vi "总磷氨氮测量流程.vi"(10 "量程模式":T1, 11 "参数":T2={"站号"=1, "量程切换"=enum."AUTO", "控制命令"=enum."启动测量", "模式设置"=enum."待机", "测量间隔"=0} {"站号" items=["总磷"=1, "总氮"=2]}) -> ()   [LabVIEW 2016, in "斯坦道仪器.lvlib"]
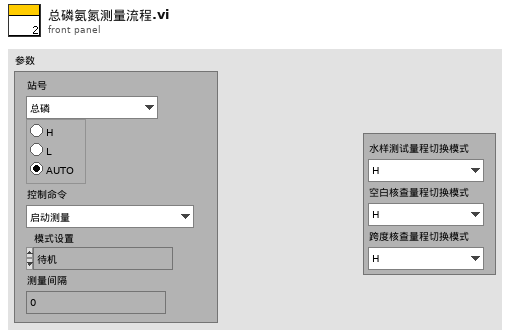
[diagram p1: front panel]
types:
  T1 = cluster{"水样测试量程切换模式":enum16{"H", "L", "AUTO"}, "空白核查量程切换模式":enum16{"H", "L", "AUTO"}, "跨度核查量程切换模式":enum16{"H", "L", "AUTO"}}
  T2 = cluster{"站号":u16, "量程切换":enum32{"H", "L", "AUTO"}, "控制命令":enum16{"启动测量", "标样核查", "零点核查", "跨度核查", "空白测试", "平行样测试", "加标回收", "空白校准", "标样校准", "初始化（清洗）", "停止测试", "仪器重启", "校时", "模式设置", "测量间隔设置"}, "模式设置":enum16{"待机", "连续模式", "周期模式", "定点模式", "受控模式", "手动模式"}, "测量间隔":u16}
  T3 = enum16{"初始化", "通电", "参数1启动", "等待参数1测试完成", "参数1测试完成", "参数1存储数据", "参数2启动", "等待参数2测试完成", "参数2测试完成", "参数2存储数据", "断电", "结束"}
  T4 = cluster{"时间标识":timestamp, "设备":string, "日志信息":string, "流程参数":string}
  T5 = cluster{"时间标识":timestamp, "监测值":sgl, "单位":u16, "数据标识":string, "因子编码":u32, "标样参考值":sgl, "F0":sgl, "F1":sgl, "F2":sgl, "F3":sgl, "F4":sgl, "F5":sgl, "F6":sgl, "F7":sgl, "X":sgl, "温度":sgl, "湿度":sgl, "量程标识":string}
  T6 = enum16{"维护数据", "水样测试", "标样核查", "零点核查", "跨度核查", "空白测试", "平行样测试", "加标回收", "空白校准", "标样校准", "初始化（清洗）"}
  T7 = cluster{"系统时间":timestamp, "工作状态":enum16{"空闲", "水样测试", "标样核查", "零点核查", "跨度核查", "空白测试", "平行样测试", "加标回收", "空白校准", "标样校准", "初始化（清洗）"}, "测量模式":enum16{"待机", "连续模式", "周期模式", "定点模式", "受控模式", "手动模式"}, "告警代码":enum16{"无告警", "缺试剂告警", "缺水样告警", "缺蒸馏水告警", "缺标液告警", "仪表漏液告警", "标定异常告警", "超量程告警", "加热异常", "低试剂预警", "超上限告警", "超下限告警", "仪表内部其他异常", "滴定异常告警", "电极异常告警", "量程切换告警", "参数设置告警", "PH电极电位异常", "电导率电极异常", "浊度光度异常", "溶解氧电极异常", "溶解氧光强异常", "温度异常告警", "PH异常告警", "溶解氧异常告警", "电导率异常告警", "浊度异常告警", "叶绿素异常告警", "藻密度异常告警", "蓝绿藻异常告警", "ORP异常告警", "氨氮异常告警", "清洁刷异常告警", "SD卡异常告警", "蓝牙异常告警", "Wifi异常告警", "流程异常告警"}, "故障代码":enum16{"无故障", "电机故障", "温度故障", "通讯故障", "滴定故障"}, "日志代码":u16, "软件版本":u16, "F0":sgl, "F1":sgl, "F2":sgl, "F3":sgl, "T":sgl, "H":sgl, "id":u16, "flowid":u16, "量程":u16}
  T8 = enum16{"启动测量", "标样核查", "零点核查", "跨度核查", "空白测试", "平行样测试", "加标回收", "空白校准", "标样校准", "初始化（清洗）", "停止测试", "仪器重启", "校时", "模式设置", "测量间隔设置"}
  T9 = enum16{"空闲", "水样测试", "标样核查", "零点核查", "跨度核查", "空白测试", "平行样测试", "加标回收", "空白校准", "标样校准", "初始化（清洗）"}
  T10 = cluster{"时间标识":timestamp, "监测值":sgl, "单位":u16, "数据标识":string, "因子编码":u32, "标样参考值":sgl, "F0":sgl, "F1":sgl, "F2":sgl, "F3":sgl, "温度":sgl, "湿度":sgl, "量程标识":string}
  T11 = cluster{"因子编码":u32, "单位":u16, "标样参考值":sgl, "水样数据时间":timestamp, "水样实测值":sgl, "水样数据标识":string, "标样数据时间":timestamp, "标样实测值":sgl, "标样数据标识":string, "空白数据时间":timestamp, "空白实测值":sgl, "空白数据标识":string, "零点核查数据时间":timestamp, "零点核查实测值":sgl, "零点核查数据标识":string, "跨度核查数据时间":timestamp, "跨度核查实测值":sgl, "跨度核查数据标识":string, "加标回收数据时间":timestamp, "加标回收实测值":sgl, "加标回收数据标识":string, "平行样数据时间":timestamp, "平行样实测值":sgl, "平行样数据标识":string, "F0":sgl, "F1":sgl, "F2":sgl, "F3":sgl, "F4":sgl, "F5":sgl, "F6":sgl, "F7":sgl, "温度":sgl, "湿度":sgl, "X值":sgl}
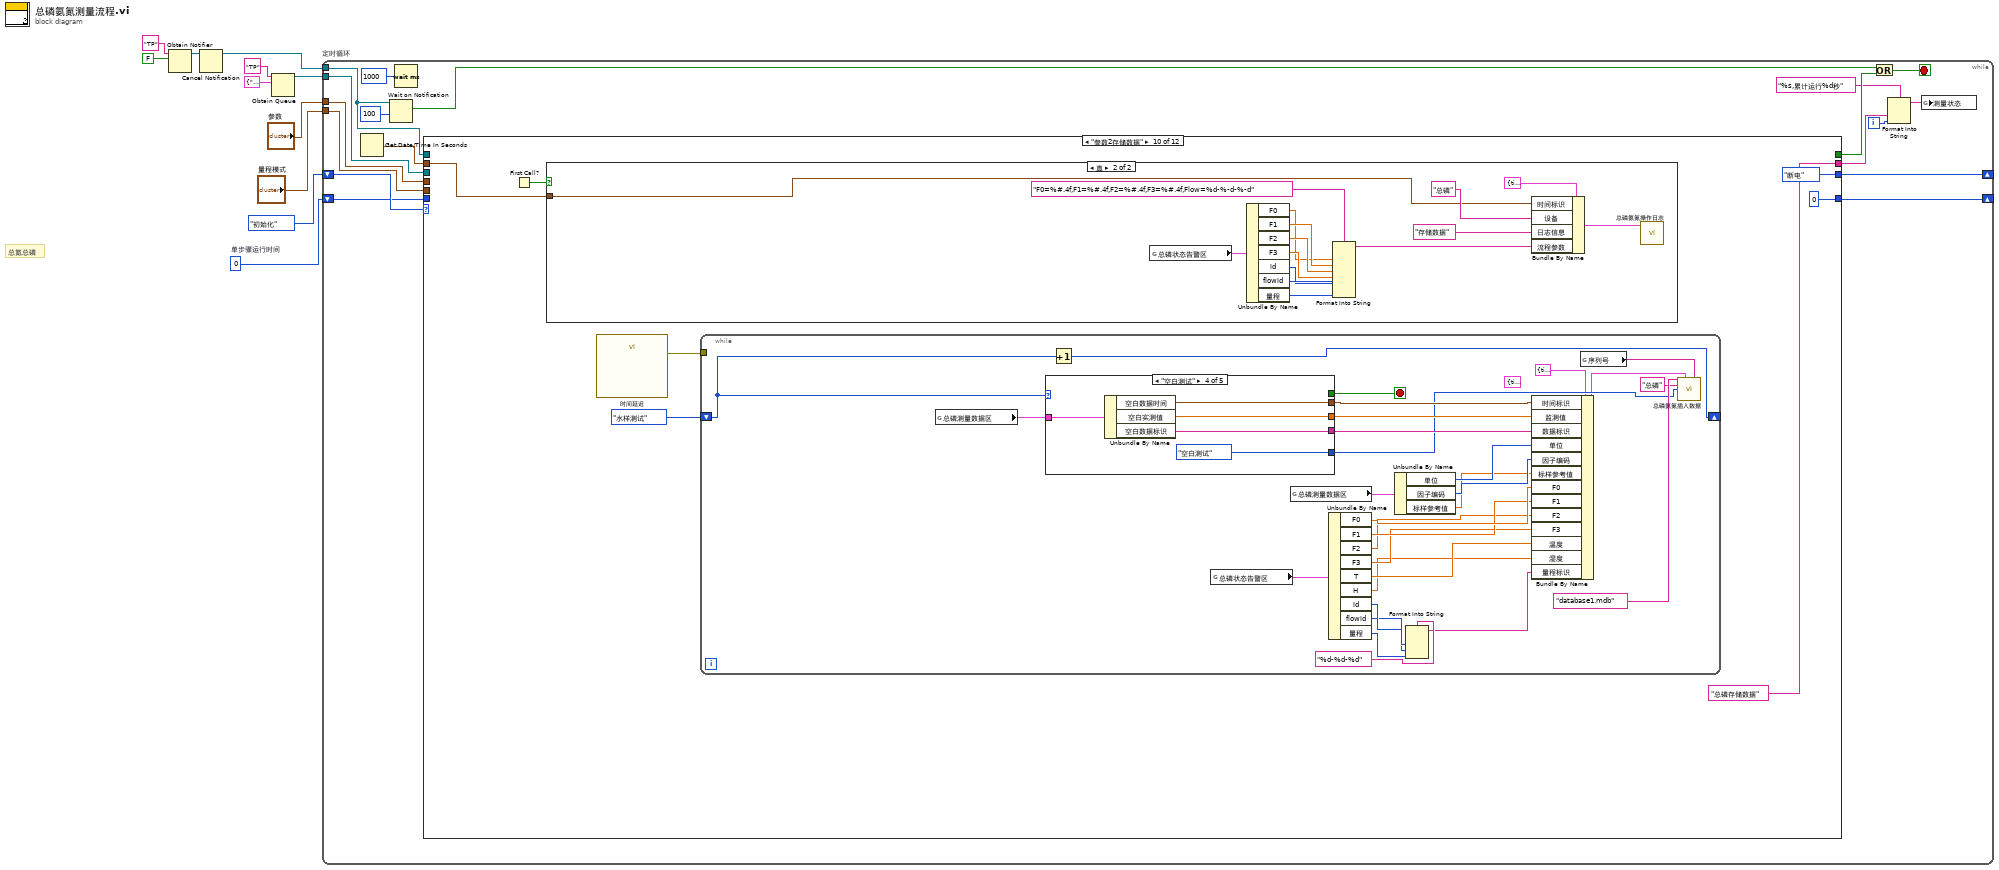
[diagram p0: block diagram]
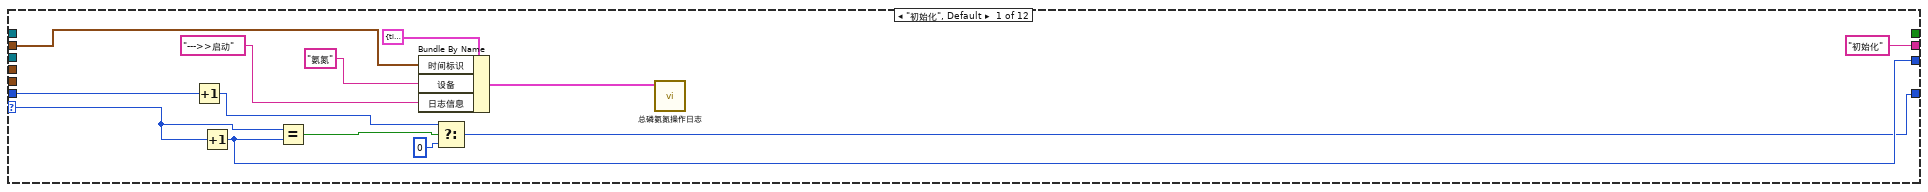
[diagram p2: hidden frame]
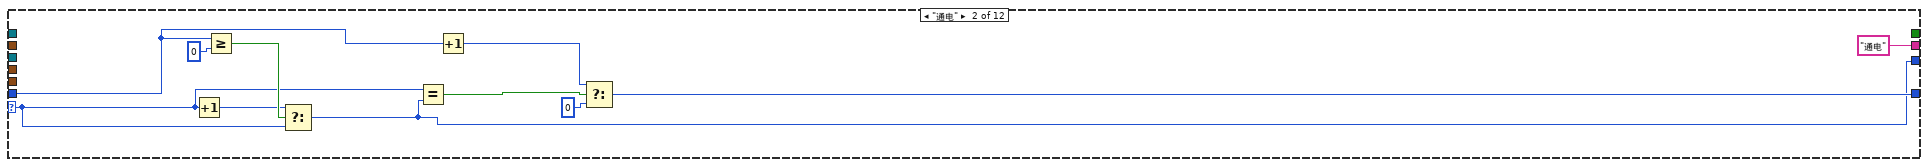
[diagram p3: hidden frame]
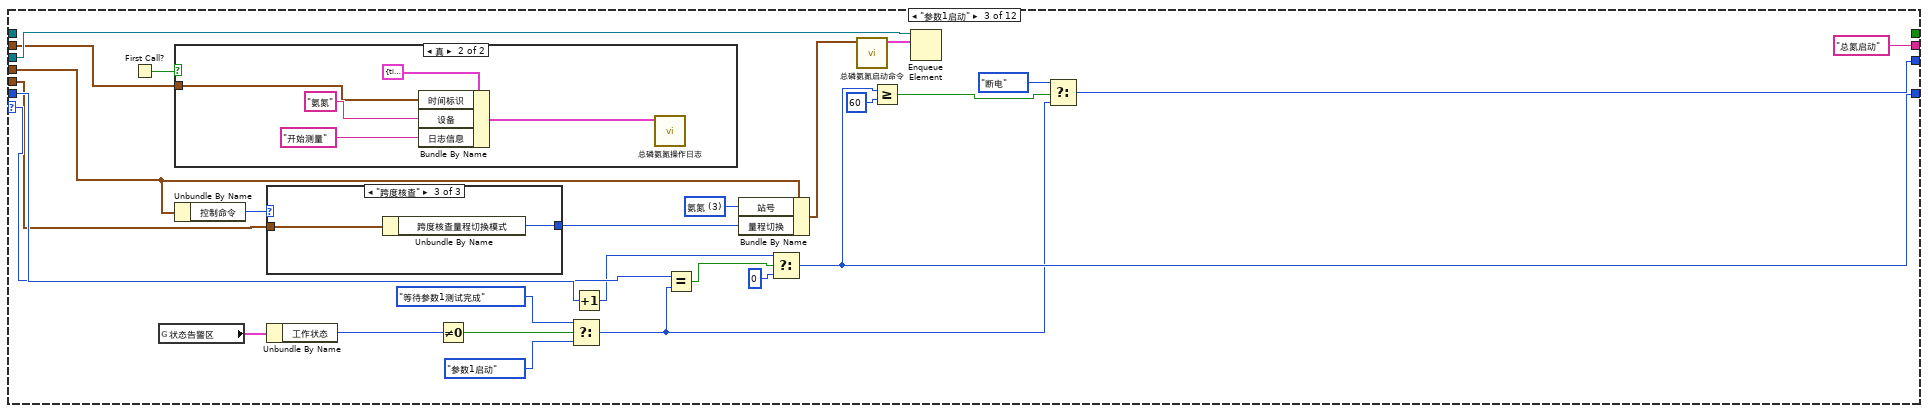
[diagram p4: hidden frame]
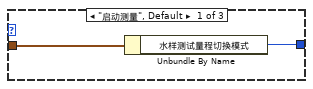
[diagram p5: hidden frame]
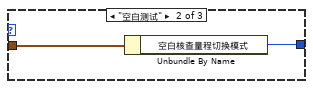
[diagram p6: hidden frame]
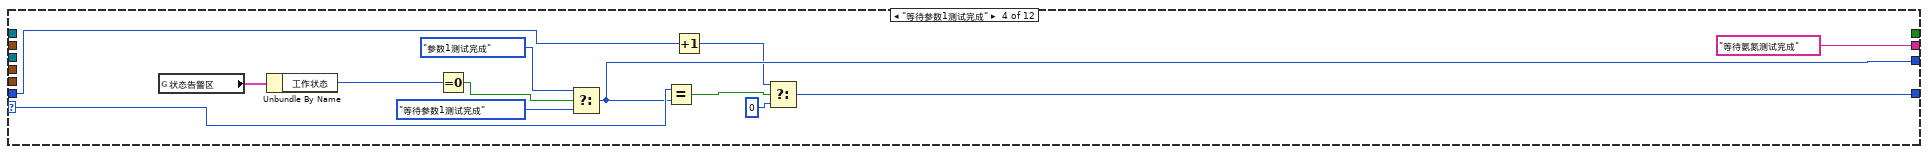
[diagram p8: hidden frame]
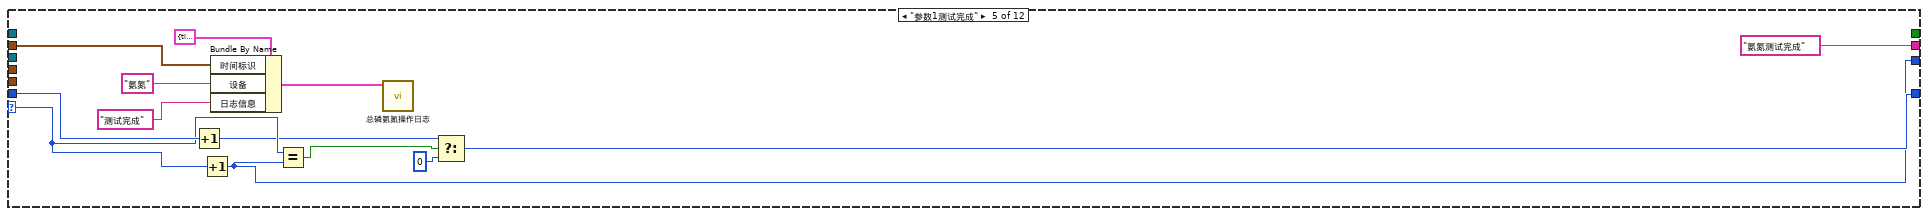
[diagram p9: hidden frame]
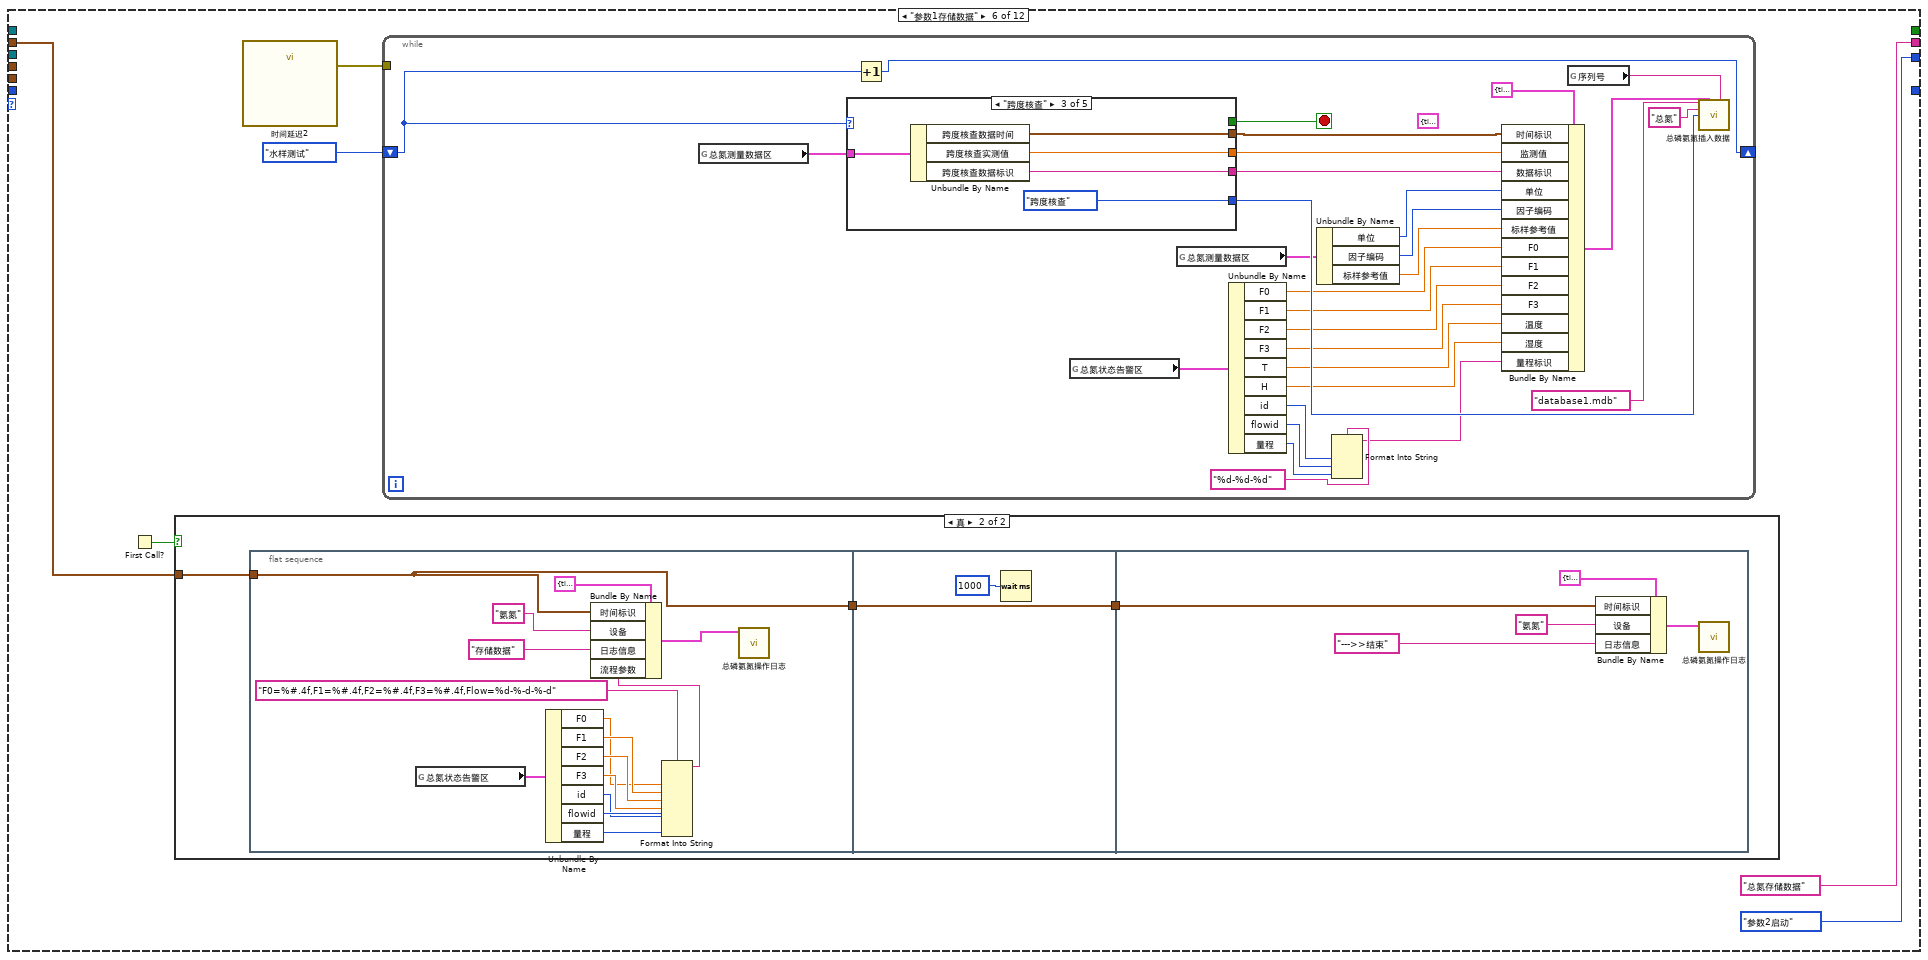
[diagram p10: hidden frame]
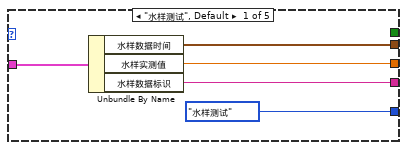
[diagram p11: hidden frame]
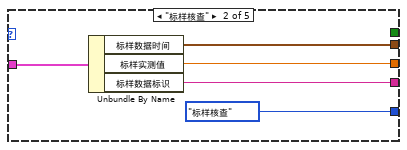
[diagram p12: hidden frame]
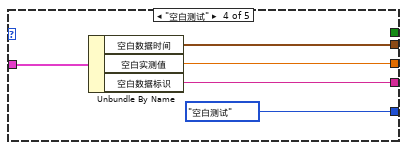
[diagram p13: hidden frame]
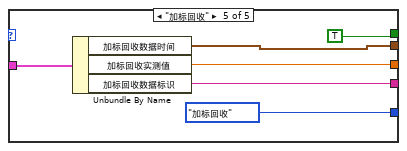
[diagram p14: hidden frame]
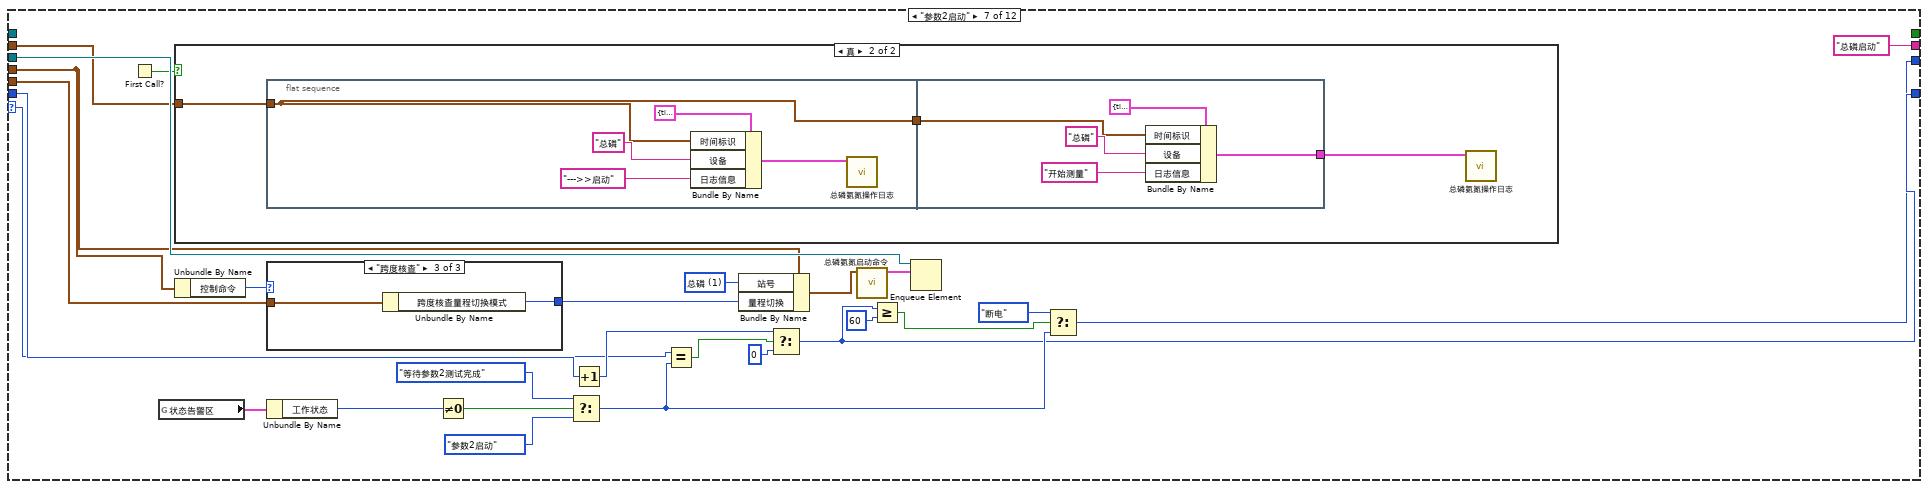
[diagram p16: hidden frame]
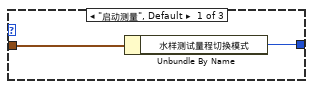
[diagram p17: hidden frame]
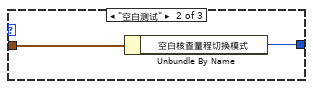
[diagram p18: hidden frame]
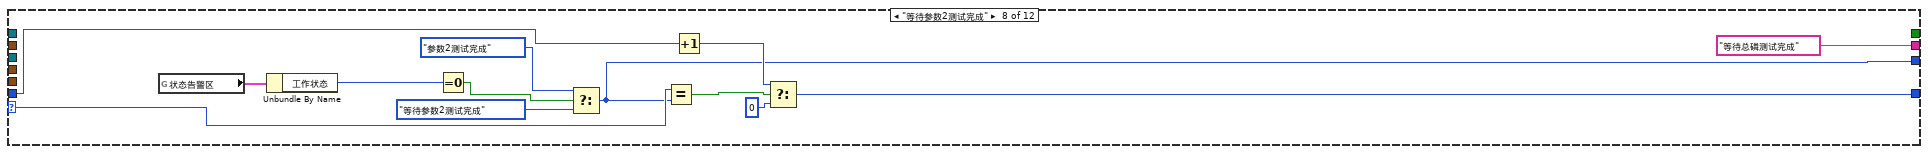
[diagram p20: hidden frame]
diagram:
  w7 = 0  # 单步骤运行时间
  # "总氮总磷"
  n1 = Obtain Notifier(name (unnamed)="TP" ("名称（未命名）"), notification data type=FALSE) -> (notifier out=w4:refnum<notifier>)  [unwired: 2 in, 2 out]
  n2 = Cancel Notification(0:w4) -> (8:w3:refnum<notifier>)  [unwired: 1 in, 2 out]
  n3 = Obtain Queue(name (unnamed)="TP" ("名称（未命名）"), element data type=cluster{"命令":string, "data":variant} {"命令"="", "data"=variant}) -> (queue out=w8:refnum<queue>)  [unwired: 3 in, 2 out]
  n4 = while "定时循环" {
    shift-right: [w28] -> _
    shift-left: T3."初始化" ("枚举") -> [w29]
    tunnel: w8 -> [w27]
    shift-right: [w25] -> _
    shift-left: w7 -> [w26]
    tunnel: w3 -> [w24]
    tunnel: "参数" -> [w19]
    tunnel: "量程模式" -> [w13]
    i -> [w15]
    stop <- w20 stop-if-true
    n5 = Get Date/Time In Seconds() -> (seconds since 1Jan1904=w17:timestamp)
    n6 = Wait on Notification(notifier=w24, timeout in ms (-1)=100 ("超时毫秒(-1)")) -> (notification=w21:bool)  [unwired: 2 in, 3 out]
    n7 = Wait (ms)(milliseconds to wait=u32 1000 ("等待时间（毫秒）")) -> ()  [unwired: 1 out]
    n8 = case shown="\"参数2存储数据\"" w29 {
      selector: w29 -> [w40 w47 w75 w99 w114 _ w219 w255 w271 _ w358 _]
      tunnel: [_ _ _ _ _ _ _ _ _ _ _ TRUE] -> w22
      tunnel: [w41 w46 w54 w98 w113 T3."参数2启动" ("枚举") w204 w253 w269 T3."断电" ("枚举") w357 T3."结束" ("枚举")] -> w28
      tunnel: w27 -> [_ _ w80 _ _ _ w227 _ _ _ _ w370]
      tunnel: w26 -> [w42 w48 w76 w101 w115 _ w220 w256 w272 _ w360 _]
      tunnel: [w38 w49 w59 w100 w116 _ w205 w254 w270 0 ("t") w359 0 ("t")] -> w25
      tunnel: w24 -> [_ _ _ _ _ _ _ _ _ _ _ w369]
      tunnel: w19 -> [_ _ w63 _ _ _ w213 _ _ _ _ _]
      tunnel: w17 -> [w31 _ w68 _ w106 w123 w218 _ w264 w281 _ w363]
      tunnel: ["初始化" ("输入 1") "通电" ("输入 1") "总氮启动" ("输入 1") "等待氨氮测试完成" ("输入 1") "氨氮测试完成" ("输入 1") "总氮存储数据" ("输入 1") "总磷启动" ("输入 1") "等待总磷测试完成" ("输入 1") "总磷测试完成" ("输入 1") "总磷存储数据" ("输入 1") "断电" ("输入 1") "结束" ("输入 1")] -> w14
      tunnel: w13 -> [_ _ w61 _ _ _ w211 _ _ _ _ _]
      frame "初始化", Default {
        n9 = Increment(x=w42) -> (x+1=w36:i32)
        n10 = Increment(x=w40) -> (x+1=w41:T3)
        n11 = Equal?(x=w40, y=w41) -> (x = y?=w39:bool)
        n12 = Bundle By Name(cluster=T4 {"时间标识"=timestamp(0 s since 1904-01-01), "设备"="", "日志信息"="", "流程参数"=""} ("data in"), "时间标识"=w31, "设备"="氨氮", "日志信息"="--->>启动") -> (w35:T4)
        n13 = Select(t=w36, s=w39, f=0 ("t")) -> (s? t:f=w38:i32)
        n14 = call "总磷氨氮操作日志.vi"("data in"=w35) -> ()  [unwired: 11 in]
      }
      frame "通电" {
        n15 = Increment(x=w47) -> (x+1=w51:T3)
        n16 = Greater Or Equal?(x=w48, y=0) -> (x >= y?=w52:bool)
        n17 = Select(t=w51, s=w52, f=w47) -> (s? t:f=w46:T3)
        n18 = Equal?(x=w47, y=w46) -> (x = y?=w50:bool)
        n19 = Increment(x=w48) -> (x+1=w45:i32)
        n20 = Select(t=w45, s=w50, f=0 ("t")) -> (s? t:f=w49:i32)
      }
      frame "参数1启动" {
        w70 = u16 3 items=["总磷"=1, "总氮"=2, "氨氮"=3] ("站号")
        n21 = First Call?() -> (First Call?: T/F=w67:bool)
        n22 = global read "VAR总磷氨氮全局变量.vi" "状态告警区"() -> (w69:T7)
        n23 = case shown="真" w67 {
          tunnel: w68 -> [_ w87]
          frame False {
          }
          frame True {
            n24 = Bundle By Name(cluster=T4 {"时间标识"=timestamp(0 s since 1904-01-01), "设备"="", "日志信息"="", "流程参数"=""} ("data in"), "时间标识"=w87, "设备"="氨氮", "日志信息"="开始测量") -> (w91:T4)
            n25 = call "总磷氨氮操作日志.vi"("data in"=w91) -> ()  [unwired: 11 in]
          }
        }
        n26 = Unbundle By Name(w63) -> ("控制命令"=w62:T8)
        n27 = case shown="\"跨度核查\"" w62 {
          tunnel: w61 -> [w82 w84 w86]
          tunnel: [w81 w83 w85] -> w60
          frame "启动测量", Default {
            n28 = Unbundle By Name(w82) -> ("水样测试量程切换模式"=w81:enum16{"H", "L", "AUTO"})
          }
          frame "空白测试" {
            n29 = Unbundle By Name(w84) -> ("空白核查量程切换模式"=w83:enum16{"H", "L", "AUTO"})
          }
          frame "跨度核查" {
            n30 = Unbundle By Name(w86) -> ("跨度核查量程切换模式"=w85:enum16{"H", "L", "AUTO"})
          }
        }
        n31 = Unbundle By Name(w69) -> ("工作状态"=w79:T9)
        n32 = Not Equal To 0?(x=w79) -> (x != 0?=w78:bool)
        n33 = Select(t=T3."等待参数1测试完成" ("枚举"), s=w78, f=T3."参数1启动" ("枚举")) -> (s? t:f=w56:T3)
        n34 = Increment(x=w76) -> (x+1=w73:i32)
        n35 = Equal?(x=w75, y=w56) -> (x = y?=w77:bool)
        n36 = Bundle By Name(cluster=w63, "站号"=w70, "量程切换"=w60) -> (w71:T2)
        n37 = Select(t=w73, s=w77, f=0 ("t")) -> (s? t:f=w59:i32)
        n38 = call "总磷氨氮启动命令.vi"("参数"=w71) -> ("启动命令"=w72:cluster{"命令":string, "data":variant})  [unwired: 10 in]
        n39 = Greater Or Equal?(x=w59, y=60) -> (x >= y?=w57:bool)
        n40 = Enqueue Element(queue=w80, element=w72) -> ()  [unwired: 2 in, 3 out]
        n41 = Select(t=T3."断电" ("枚举"), s=w57, f=w56) -> (s? t:f=w54:T3)
      }
      frame "等待参数1测试完成" {
        n42 = global read "VAR总磷氨氮全局变量.vi" "状态告警区"() -> (w95:T7)
        n43 = Unbundle By Name(w95) -> ("工作状态"=w104:T9)
        n44 = Equal To 0?(x=w104) -> (x = 0?=w103:bool)
        n45 = Select(t=T3."参数1测试完成" ("枚举"), s=w103, f=T3."等待参数1测试完成" ("枚举")) -> (s? t:f=w98:T3)
        n46 = Equal?(x=w99, y=w98) -> (x = y?=w102:bool)
        n47 = Increment(x=w101) -> (x+1=w96:i32)
        n48 = Select(t=w96, s=w102, f=0 ("t")) -> (s? t:f=w100:i32)
      }
      frame "参数1测试完成" {
        n49 = Increment(x=w115) -> (x+1=w111:i32)
        n50 = Increment(x=w114) -> (x+1=w113:T3)
        n51 = Bundle By Name(cluster=T4 {"时间标识"=timestamp(0 s since 1904-01-01), "设备"="", "日志信息"="", "流程参数"=""} ("data in"), "时间标识"=w106, "设备"="氨氮", "日志信息"="测试完成") -> (w110:T4)
        n52 = Equal?(x=w114, y=w113) -> (x = y?=w117:bool)
        n53 = call "总磷氨氮操作日志.vi"("data in"=w110) -> ()  [unwired: 11 in]
        n54 = Select(t=w111, s=w117, f=0 ("t")) -> (s? t:f=w116:i32)
      }
      frame "参数1存储数据" {
        n55 = First Call?() -> (First Call?: T/F=w121:bool)
        n56 = case shown="真" w121 {
          tunnel: w123 -> [_ w181]
          frame False {
          }
          frame True {
            n57 = flat-sequence {
              tunnel: w181 -> [w192]
              tunnel: [w192] -> w180
              tunnel: w180 -> [w198]
              tunnel: [w198] -> w179
              tunnel: w179 -> [w199]
              frame #0 {
                n58 = global read "VAR总磷氨氮全局变量.vi" "总氮状态告警区"() -> (w191:T7)
                n59 = Unbundle By Name(w191) -> ("F0"=w183:sgl, "F1"=w184:sgl, "F2"=w185:sgl, "F3"=w186:sgl, "id"=w187:u16, "flowid"=w188:u16, "量程"=w189:u16)
                n60 = Format Into String(format string="F0=%#.4f,F1=%#.4f,F2=%#.4f,F3=%#.4f,Flow=%d-%-d-%-d" ("格式字符串"), w183, w184, w185, w186, w187, w188, w189) -> (resulting string=w182:string)  [unwired: 2 in, 1 out]
                n61 = Bundle By Name(cluster=T4 {"时间标识"=timestamp(0 s since 1904-01-01), "设备"="", "日志信息"="", "流程参数"=""} ("data in"), "时间标识"=w192, "设备"="氨氮", "日志信息"="存储数据", "流程参数"=w182) -> (w196:T4)
                n62 = call "总磷氨氮操作日志.vi"("data in"=w196) -> ()  [unwired: 11 in]
              }
              frame #1 {
                n63 = Wait (ms)(milliseconds to wait=u32 1000 ("等待时间（毫秒）")) -> ()  [unwired: 1 out]
              }
              frame #2 {
                n64 = Bundle By Name(cluster=T4 {"时间标识"=timestamp(0 s since 1904-01-01), "设备"="", "日志信息"="", "流程参数"=""} ("data in"), "时间标识"=w199, "设备"="氨氮", "日志信息"="--->>结束") -> (w200:T4)
                n65 = call "总磷氨氮操作日志.vi"("data in"=w200) -> ()  [unwired: 11 in]
              }
            }
          }
        }
        n66 = call "时间延迟2"() -> ("error out"=w118:errorcluster)  [unwired: 11 in]
        n67 = while {
          shift-right: [w140] -> _
          shift-left: enum16{"水样测试", "标样核查", "跨度核查", "空白测试", "加标回收"}."水样测试" ("测量模式") -> [w141]
          tunnel: w118 -> [_]
          stop <- w142 stop-if-true
          (unwired) T10 {"时间标识"=timestamp(0 s since 1904-01-01), "监测值"=0.0, "单位"=0, "数据标识"="", "因子编码"=0, "标样参考值"=0.0, "F0"=0.0, "F1"=0.0, "F2"=0.0, "F3"=0.0, "温度"=0.0, "湿度"=0.0, "量程标识"=""} ("data")
          n68 = global read "VAR总磷氨氮全局变量.vi" "总氮测量数据区"() -> (w144:T11)
          n69 = case shown="\"跨度核查\"" w141 {
            tunnel: w144 -> [w153 w158 w163 w168 w173]
            tunnel: [w157 w162 w167 w172 w178] -> w137
            tunnel: [w156 w161 w166 w171 w177] -> w136
            tunnel: [w155 w160 w165 w170 w176] -> w135
            tunnel: [T6."水样测试" ("测量模式") T6."标样核查" ("测量模式") T6."跨度核查" ("测量模式") T6."空白测试" ("测量模式") T6."加标回收" ("测量模式")] -> w143
            tunnel: [_ _ _ _ TRUE] -> w142
            frame "水样测试", Default {
              n70 = Unbundle By Name(w153) -> ("水样数据时间"=w157:timestamp, "水样实测值"=w156:sgl, "水样数据标识"=w155:string)
            }
            frame "标样核查" {
              n71 = Unbundle By Name(w158) -> ("标样数据时间"=w162:timestamp, "标样实测值"=w161:sgl, "标样数据标识"=w160:string)
            }
            frame "跨度核查" {
              n72 = Unbundle By Name(w163) -> ("跨度核查数据时间"=w167:timestamp, "跨度核查实测值"=w166:sgl, "跨度核查数据标识"=w165:string)
            }
            frame "空白测试" {
              n73 = Unbundle By Name(w168) -> ("空白数据时间"=w172:timestamp, "空白实测值"=w171:sgl, "空白数据标识"=w170:string)
            }
            frame "加标回收" {
              n74 = Unbundle By Name(w173) -> ("加标回收数据时间"=w178:timestamp, "加标回收实测值"=w177:sgl, "加标回收数据标识"=w176:string)
            }
          }
          n75 = Increment(x=w141) -> (x+1=w140:enum16{"水样测试", "标样核查", "跨度核查", "空白测试", "加标回收"})
          n76 = global read "VAR总磷氨氮全局变量.vi" "总氮状态告警区"() -> (w152:T7)
          n77 = global read "VAR总磷氨氮全局变量.vi" "总氮测量数据区"() -> (w139:T11)
          n78 = Unbundle By Name(w152) -> ("F0"=w131:sgl, "F1"=w130:sgl, "F2"=w129:sgl, "F3"=w128:sgl, "T"=w127:sgl, "H"=w126:sgl, "id"=w148:u16, "flowid"=w147:u16, "量程"=w146:u16)
          n79 = Unbundle By Name(w139) -> ("单位"=w134:u16, "因子编码"=w133:u32, "标样参考值"=w132:sgl)
          n80 = Format Into String(format string="%d-%d-%d" ("格式字符串"), w148, w147, w146) -> (resulting string=w138:string)  [unwired: 2 in, 1 out]
          n81 = Bundle By Name(cluster=T5 {"时间标识"=timestamp(0 s since 1904-01-01), "监测值"=0.0, "单位"=0, "数据标识"="", "因子编码"=0, "标样参考值"=0.0, "F0"=0.0, "F1"=0.0, "F2"=0.0, "F3"=0.0, "F4"=0.0, "F5"=0.0, "F6"=0.0, "F7"=0.0, "X"=0.0, "温度"=0.0, "湿度"=0.0, "量程标识"=""} ("data"), "时间标识"=w137, "监测值"=w136, "数据标识"=w135, "单位"=w134, "因子编码"=w133, "标样参考值"=w132, "F0"=w131, "F1"=w130, "F2"=w129, "F3"=w128, "温度"=w127, "湿度"=w126, "量程标识"=w138) -> (w124:T5)
          n82 = global read "VAR总磷氨氮全局变量.vi" "序列号"() -> (w145:string)
          n83 = call "总磷氨氮插入数据.vi"("database"="database1.mdb", "data"=w124, "SN"=w145, "table"="总氮", "测量模式"=w143) -> ()  [unwired: 10 in, 1 out]
        }
      }
      frame "参数2启动" {
        w228 = u16 1 items=["总氮"=2, "总磷"=1] ("站号")
        n84 = First Call?() -> (First Call?: T/F=w217:bool)
        n85 = global read "VAR总磷氨氮全局变量.vi" "状态告警区"() -> (w221:T7)
        n86 = case shown="真" w217 {
          tunnel: w218 -> [_ w237]
          frame False {
          }
          frame True {
            n87 = flat-sequence {
              tunnel: w237 -> [w240]
              tunnel: [w240] -> w238
              tunnel: [w249] -> w239
              tunnel: w238 -> [w245]
              frame #0 {
                n88 = Bundle By Name(cluster=T4 {"时间标识"=timestamp(0 s since 1904-01-01), "设备"="", "日志信息"="", "流程参数"=""} ("data in"), "时间标识"=w240, "设备"="总磷", "日志信息"="--->>启动") -> (w244:T4)
                n89 = call "总磷氨氮操作日志.vi"("data in"=w244) -> ()  [unwired: 11 in]
              }
              frame #1 {
                n90 = Bundle By Name(cluster=T4 {"时间标识"=timestamp(0 s since 1904-01-01), "设备"="", "日志信息"="", "流程参数"=""} ("data in"), "时间标识"=w245, "设备"="总磷", "日志信息"="开始测量") -> (w249:T4)
              }
            }
            n91 = call "总磷氨氮操作日志.vi"("data in"=w239) -> ()  [unwired: 11 in]
          }
        }
        n92 = Unbundle By Name(w213) -> ("控制命令"=w212:T8)
        n93 = case shown="\"跨度核查\"" w212 {
          tunnel: w211 -> [w232 w234 w236]
          tunnel: [w231 w233 w235] -> w210
          frame "启动测量", Default {
            n94 = Unbundle By Name(w232) -> ("水样测试量程切换模式"=w231:enum16{"H", "L", "AUTO"})
          }
          frame "空白测试" {
            n95 = Unbundle By Name(w234) -> ("空白核查量程切换模式"=w233:enum16{"H", "L", "AUTO"})
          }
          frame "跨度核查" {
            n96 = Unbundle By Name(w236) -> ("跨度核查量程切换模式"=w235:enum16{"H", "L", "AUTO"})
          }
        }
        n97 = Unbundle By Name(w221) -> ("工作状态"=w226:T9)
        n98 = Not Equal To 0?(x=w226) -> (x != 0?=w225:bool)
        n99 = Select(t=T3."等待参数2测试完成" ("枚举"), s=w225, f=T3."参数2启动" ("枚举")) -> (s? t:f=w206:T3)
        n100 = Increment(x=w220) -> (x+1=w222:i32)
        n101 = Equal?(x=w219, y=w206) -> (x = y?=w224:bool)
        n102 = Bundle By Name(cluster=w213, "站号"=w228, "量程切换"=w210) -> (w229:T2)
        n103 = Select(t=w222, s=w224, f=0 ("t")) -> (s? t:f=w205:i32)
        n104 = call "总磷氨氮启动命令.vi"("参数"=w229) -> ("启动命令"=w230:cluster{"命令":string, "data":variant})  [unwired: 10 in]
        n105 = Greater Or Equal?(x=w205, y=60) -> (x >= y?=w208:bool)
        n106 = Enqueue Element(queue=w227, element=w230) -> ()  [unwired: 2 in, 3 out]
        n107 = Select(t=T3."断电" ("枚举"), s=w208, f=w206) -> (s? t:f=w204:T3)
      }
      frame "等待参数2测试完成" {
        n108 = global read "VAR总磷氨氮全局变量.vi" "状态告警区"() -> (w257:T7)
        n109 = Unbundle By Name(w257) -> ("工作状态"=w262:T9)
        n110 = Equal To 0?(x=w262) -> (x = 0?=w261:bool)
        n111 = Select(t=T3."参数2测试完成" ("枚举"), s=w261, f=T3."等待参数2测试完成" ("枚举")) -> (s? t:f=w253:T3)
        n112 = Equal?(x=w255, y=w253) -> (x = y?=w260:bool)
        n113 = Increment(x=w256) -> (x+1=w258:i32)
        n114 = Select(t=w258, s=w260, f=0 ("t")) -> (s? t:f=w254:i32)
      }
      frame "参数2测试完成" {
        n115 = Increment(x=w272) -> (x+1=w273:i32)
        n116 = Increment(x=w271) -> (x+1=w269:T3)
        n117 = Bundle By Name(cluster=T4 {"时间标识"=timestamp(0 s since 1904-01-01), "设备"="", "日志信息"="", "流程参数"=""} ("data in"), "时间标识"=w264, "设备"="总磷", "日志信息"="测试完成") -> (w268:T4)
        n118 = Equal?(x=w271, y=w269) -> (x = y?=w275:bool)
        n119 = call "总磷氨氮操作日志.vi"("data in"=w268) -> ()  [unwired: 11 in]
        n120 = Select(t=w273, s=w275, f=0 ("t")) -> (s? t:f=w270:i32)
      }
      frame "参数2存储数据" {
        n121 = First Call?() -> (First Call?: T/F=w278:bool)
        n122 = case shown="真" w278 {
          tunnel: w281 -> [_ w348]
          frame False {
          }
          frame True {
            n123 = global read "VAR总磷氨氮全局变量.vi" "总磷状态告警区"() -> (w347:T7)
            n124 = Unbundle By Name(w347) -> ("F0"=w339:sgl, "F1"=w340:sgl, "F2"=w341:sgl, "F3"=w342:sgl, "id"=w343:u16, "flowid"=w344:u16, "量程"=w345:u16)
            n125 = Format Into String(format string="F0=%#.4f,F1=%#.4f,F2=%#.4f,F3=%#.4f,Flow=%d-%-d-%-d" ("格式字符串"), w339, w340, w341, w342, w343, w344, w345) -> (resulting string=w338:string)  [unwired: 2 in, 1 out]
            n126 = Bundle By Name(cluster=T4 {"时间标识"=timestamp(0 s since 1904-01-01), "设备"="", "日志信息"="", "流程参数"=""} ("data in"), "时间标识"=w348, "设备"="总磷", "日志信息"="存储数据", "流程参数"=w338) -> (w352:T4)
            n127 = call "总磷氨氮操作日志.vi"("data in"=w352) -> ()  [unwired: 11 in]
          }
        }
        n128 = call "时间延迟"() -> ("error out"=w276:errorcluster)  [unwired: 11 in]
        n129 = while {
          shift-right: [w294] -> _
          shift-left: enum16{"水样测试", "标样核查", "跨度核查", "空白测试", "加标回收"}."水样测试" ("测量模式") -> [w295]
          tunnel: w276 -> [_]
          stop <- w296 stop-if-true
          (unwired) T10 {"时间标识"=timestamp(0 s since 1904-01-01), "监测值"=0.0, "单位"=0, "数据标识"="", "因子编码"=0, "标样参考值"=0.0, "F0"=0.0, "F1"=0.0, "F2"=0.0, "F3"=0.0, "温度"=0.0, "湿度"=0.0, "量程标识"=""} ("data")
          n130 = global read "VAR总磷氨氮全局变量.vi" "总磷测量数据区"() -> (w293:T11)
          n131 = case shown="\"空白测试\"" w295 {
            tunnel: w293 -> [w316 w321 w326 w331 w337]
            tunnel: [w315 w320 w325 w330 w336] -> w300
            tunnel: [w314 w319 w324 w329 w335] -> w299
            tunnel: [w313 w318 w323 w328 w334] -> w298
            tunnel: [T6."水样测试" ("测量模式") T6."标样核查" ("测量模式") T6."跨度核查" ("测量模式") T6."空白测试" ("测量模式") T6."加标回收" ("测量模式")] -> w297
            tunnel: [_ _ _ _ TRUE] -> w296
            frame "水样测试", Default {
              n132 = Unbundle By Name(w316) -> ("水样数据时间"=w315:timestamp, "水样实测值"=w314:sgl, "水样数据标识"=w313:string)
            }
            frame "标样核查" {
              n133 = Unbundle By Name(w321) -> ("标样数据时间"=w320:timestamp, "标样实测值"=w319:sgl, "标样数据标识"=w318:string)
            }
            frame "跨度核查" {
              n134 = Unbundle By Name(w326) -> ("跨度核查数据时间"=w325:timestamp, "跨度核查实测值"=w324:sgl, "跨度核查数据标识"=w323:string)
            }
            frame "空白测试" {
              n135 = Unbundle By Name(w331) -> ("空白数据时间"=w330:timestamp, "空白实测值"=w329:sgl, "空白数据标识"=w328:string)
            }
            frame "加标回收" {
              n136 = Unbundle By Name(w337) -> ("加标回收数据时间"=w336:timestamp, "加标回收实测值"=w335:sgl, "加标回收数据标识"=w334:string)
            }
          }
          n137 = Increment(x=w295) -> (x+1=w294:enum16{"水样测试", "标样核查", "跨度核查", "空白测试", "加标回收"})
          n138 = global read "VAR总磷氨氮全局变量.vi" "总磷状态告警区"() -> (w308:T7)
          n139 = global read "VAR总磷氨氮全局变量.vi" "总磷测量数据区"() -> (w292:T11)
          n140 = Unbundle By Name(w308) -> ("F0"=w289:sgl, "F1"=w288:sgl, "F2"=w287:sgl, "F3"=w286:sgl, "T"=w285:sgl, "H"=w284:sgl, "id"=w304:u16, "flowid"=w303:u16, "量程"=w302:u16)
          n141 = Unbundle By Name(w292) -> ("单位"=w311:u16, "因子编码"=w310:u32, "标样参考值"=w309:sgl)
          n142 = Format Into String(format string="%d-%d-%d" ("格式字符串"), w304, w303, w302) -> (resulting string=w290:string)  [unwired: 2 in, 1 out]
          n143 = Bundle By Name(cluster=T5 {"时间标识"=timestamp(0 s since 1904-01-01), "监测值"=0.0, "单位"=0, "数据标识"="", "因子编码"=0, "标样参考值"=0.0, "F0"=0.0, "F1"=0.0, "F2"=0.0, "F3"=0.0, "F4"=0.0, "F5"=0.0, "F6"=0.0, "F7"=0.0, "X"=0.0, "温度"=0.0, "湿度"=0.0, "量程标识"=""} ("data"), "时间标识"=w300, "监测值"=w299, "数据标识"=w298, "单位"=w311, "因子编码"=w310, "标样参考值"=w309, "F0"=w289, "F1"=w288, "F2"=w287, "F3"=w286, "温度"=w285, "湿度"=w284, "量程标识"=w290) -> (w291:T5)
          n144 = global read "VAR总磷氨氮全局变量.vi" "序列号"() -> (w301:string)
          n145 = call "总磷氨氮插入数据.vi"("database"="database1.mdb", "data"=w291, "SN"=w301, "table"="总磷", "测量模式"=w297) -> ()  [unwired: 10 in, 1 out]
        }
      }
      frame "断电" {
        n146 = Increment(x=w360) -> (x+1=w353:i32)
        n147 = Increment(x=w358) -> (x+1=w357:T3)
        n148 = Equal?(x=w358, y=w357) -> (x = y?=w355:bool)
        n149 = Select(t=w353, s=w355, f=0 ("t")) -> (s? t:f=w359:i32)
      }
      frame "结束" {
        n150 = Release Queue(queue=w370) -> ()  [unwired: 2 in, 3 out]
        n151 = Cancel Notification(0:w369) -> (8:w368:refnum<notifier>)  [unwired: 1 in, 2 out]
        n152 = Release Notifier(notifier=w368) -> ()  [unwired: 2 in, 3 out]
        n153 = Bundle By Name(cluster=T4 {"时间标识"=timestamp(0 s since 1904-01-01), "设备"="", "日志信息"="", "流程参数"=""} ("data in"), "时间标识"=w363, "设备"="总磷", "日志信息"="--->>结束") -> (w367:T4)
        n154 = call "总磷氨氮操作日志.vi"("data in"=w367) -> ()  [unwired: 11 in]
      }
    }
    n155 = Or(x=w21, y=w22) -> (x .or. y?=w20:bool)
    n156 = Format Into String(format string="%s,累计运行%d秒" ("格式字符串"), w14, w15) -> (resulting string=w12:string)  [unwired: 2 in, 1 out]
    n157 = global write "VAR总磷氨氮全局变量.vi" "测量状态"(w12) -> ()
  }
